vi "CalcTemp.vi"(8 "error in (no error)":errorcluster, 11 "S4GUI in":refnum<class "S4GUI.lvclass">) -> (0 "error out":errorcluster, 3 "S4GUI out":refnum<class "S4GUI.lvclass">)   [LabVIEW 2018, in "S4GUI.lvclass"]
uses:
  S4GUI.lvclass
  S4GUI.lvclass/S4GUI.ctl
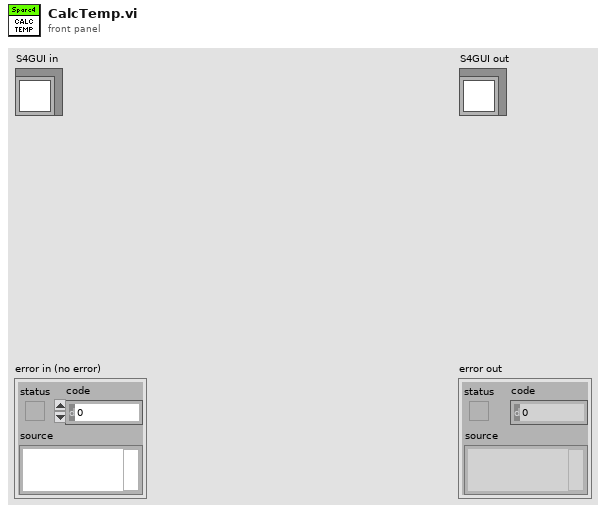
[diagram p1: front panel]
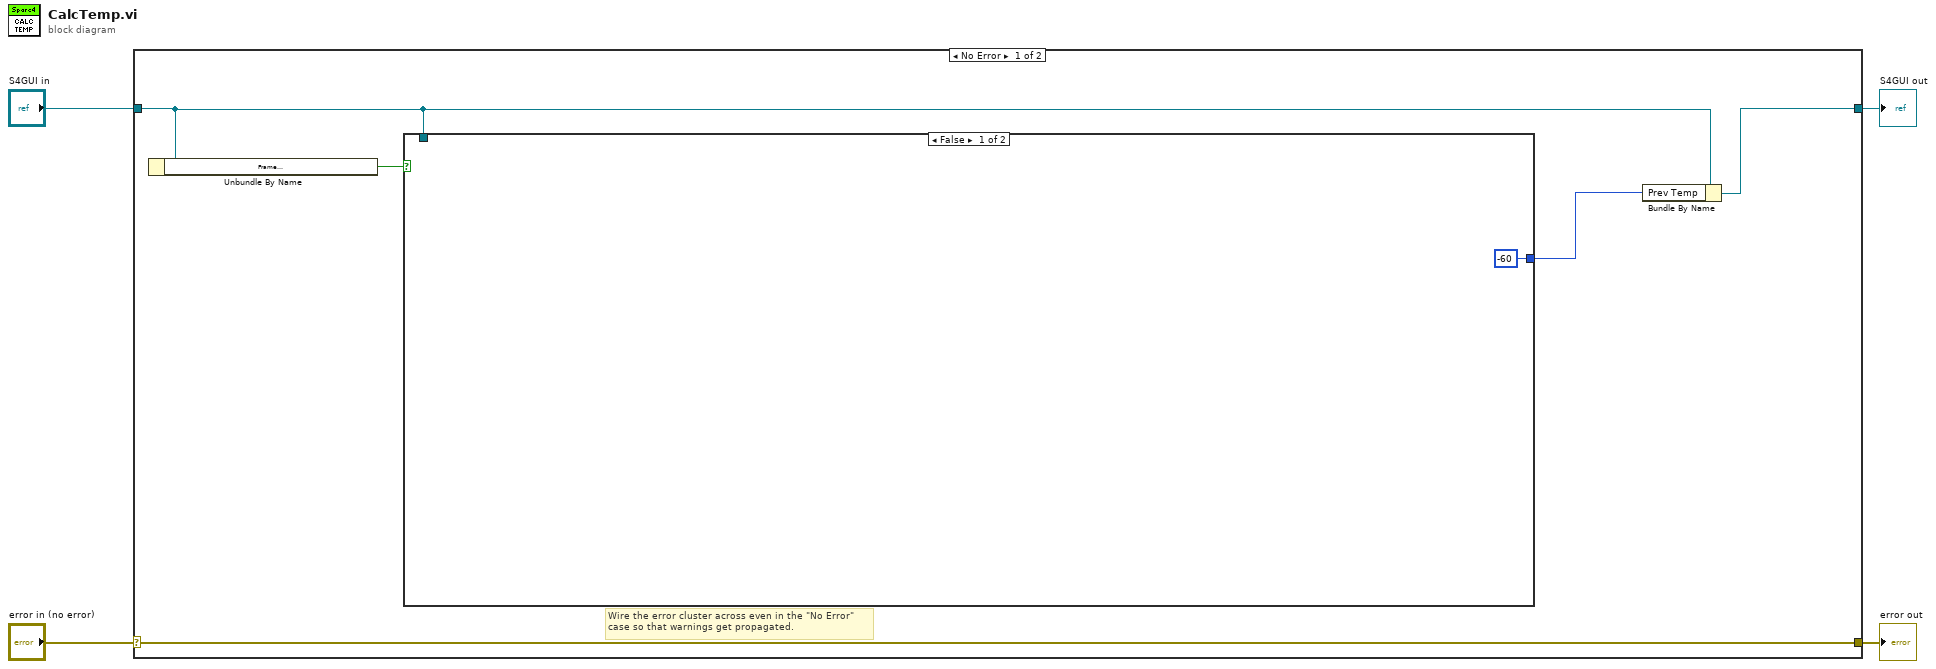
[diagram p0: block diagram]
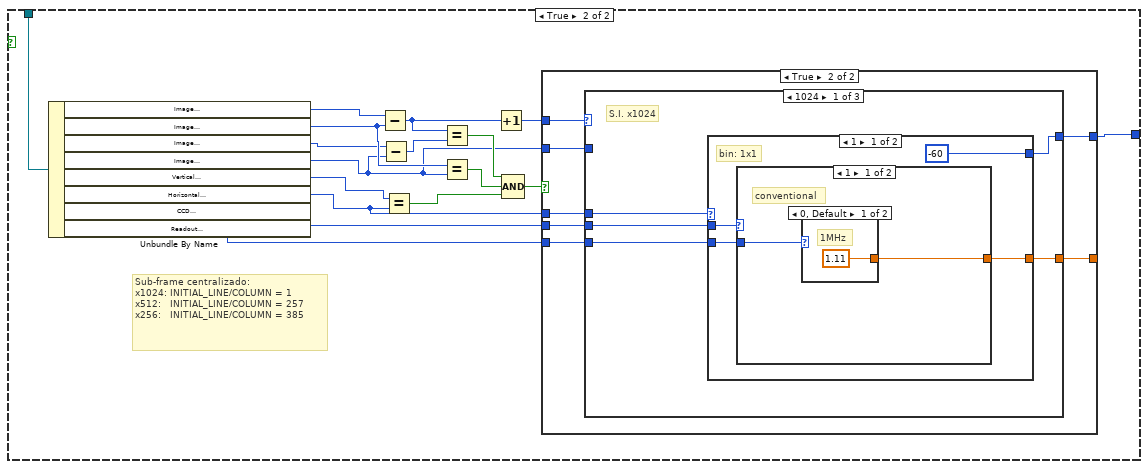
[diagram p2: hidden frame]
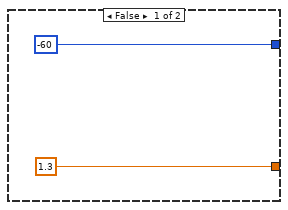
[diagram p3: hidden frame]
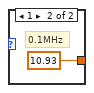
[diagram p4: hidden frame]
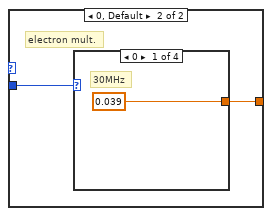
[diagram p5: hidden frame]
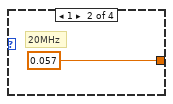
[diagram p6: hidden frame]
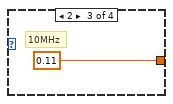
[diagram p7: hidden frame]
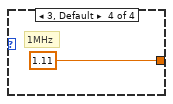
[diagram p8: hidden frame]
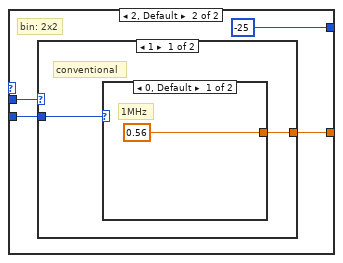
[diagram p9: hidden frame]
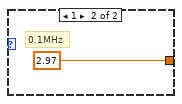
[diagram p10: hidden frame]
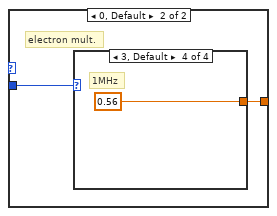
[diagram p11: hidden frame]
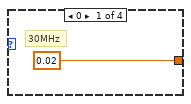
[diagram p12: hidden frame]
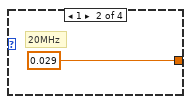
[diagram p13: hidden frame]
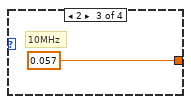
[diagram p14: hidden frame]
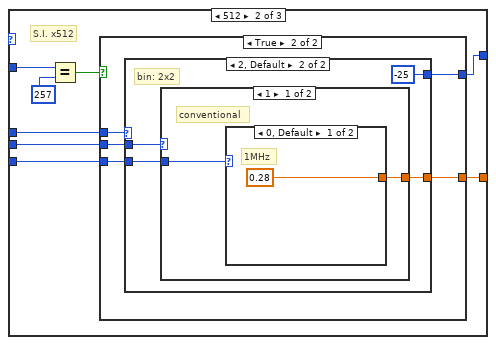
[diagram p15: hidden frame]
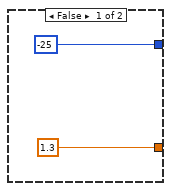
[diagram p16: hidden frame]
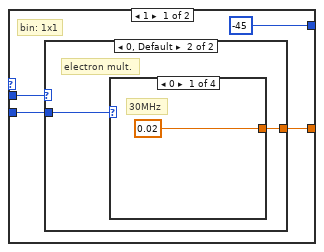
[diagram p17: hidden frame]
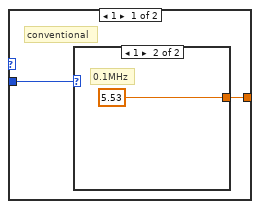
[diagram p18: hidden frame]
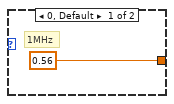
[diagram p19: hidden frame]
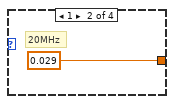
[diagram p20: hidden frame]
diagram:
  n1 = case shown="No Error" "error in (no error)" {
    selector: "error in (no error)" -> [w9 w157]
    tunnel: [w9 w157] -> w3
    tunnel: [w5 w156] -> w1
    tunnel: "S4GUI in" -> [w7 w156]
    frame No Error {
      # "Wire the error cluster across even in the \"No Error\"\ncase so that warnings get propagated."
      n2 = Unbundle By Name(w7) -> ("Frame\nTransfer"=w8:bool)
      n3 = case shown="False" w8 {
        tunnel: w7 -> [_ w27]
        tunnel: [i8 -60 ("y") w11] -> w6
        frame False {
        }
        frame True {
          # "Sub-frame centralizado:\nx1024: INITIAL_LINE/COLUMN = 1\nx512:   INITIAL_LINE/COLUMN = 257\nx256:   INITIAL_LINE/COLUMN = 385"
          n4 = Unbundle By Name(w27) -> ("Image\nFInal Column"=w19:u16, "Image\nInitial Column"=w18:u16, "Image\nFinal Line"=w17:u16, "Image \nInitial Line"=w16:u16, "Vertical\nBinning"=w15:u16, "Horizontal\nBinning"=w14:u16, "CCD \nEM Mode"=w13:u8, "Readout\nRate"=w12:u8)
          n5 = Subtract(x=w19, y=w18) -> (x-y=w23:u16)
          n6 = Subtract(x=w17, y=w16) -> (x-y=w20:u16)
          n7 = Equal?(x=w15, y=w14) -> (x = y?=w22:bool)
          n8 = Equal?(x=w23, y=w20) -> (x = y?=w25:bool)
          n9 = Equal?(x=w18, y=w16) -> (x = y?=w26:bool)
          n10 = Increment(x=w23) -> (x+1=w24:u16)
          n11 = Compound Arithmetic op=AND(w25, w26, w22) -> (w21:bool)
          n12 = case shown="True" w21 {
            tunnel: [1.3 ("y") w36] -> _
            tunnel: w13 -> [_ w35]
            tunnel: w12 -> [_ w34]
            tunnel: w24 -> [_ w33]
            tunnel: w14 -> [_ w32]
            tunnel: [i8 -60 ("y") w31] -> w11
            tunnel: w16 -> [_ w30]
            frame False {
            }
            frame True {
              n13 = case shown="1024" w33 {
                tunnel: [w41 w77 w120] -> w36
                tunnel: w35 -> [w40 w76 w119]
                tunnel: w34 -> [w39 w75 w118]
                tunnel: w32 -> [w38 w74 w117]
                tunnel: [w37 w73 w116] -> w31
                tunnel: w30 -> [_ w72 w114]
                frame 1024 {
                  # "S.I. x1024"
                  n14 = case shown="1" w38 {
                    tunnel: [w45 w59] -> w41
                    tunnel: w40 -> [w44 w58]
                    tunnel: w39 -> [w43 w57]
                    tunnel: [i8 -60 ("y") i8 -25 ("y")] -> w37
                    frame 1 {
                      # "bin: 1x1"
                      n15 = case shown="1" w44 {
                        tunnel: [w47 w51] -> w45
                        tunnel: w43 -> [w46 w50]
                        frame 1 {
                          # "conventional"
                          n16 = case shown="0, Default" w46 {
                            tunnel: [1.11 ("y") 10.93 ("y")] -> w47
                            frame 0, Default {
                              # "1MHz"
                            }
                            frame 1 {
                              # "0.1MHz"
                            }
                          }
                        }
                        frame 0, Default {
                          # "electron mult."
                          n17 = case shown="0" w50 {
                            tunnel: [0.039 ("y") 0.057 ("y") 0.11 ("y") 1.11 ("y")] -> w51
                            frame 0 {
                              # "30MHz"
                            }
                            frame 1 {
                              # "20MHz"
                            }
                            frame 2 {
                              # "10MHz"
                            }
                            frame 3, Default {
                              # "1MHz"
                            }
                          }
                        }
                      }
                    }
                    frame 2, Default {
                      # "bin: 2x2"
                      n18 = case shown="1" w58 {
                        tunnel: [w61 w65] -> w59
                        tunnel: w57 -> [w60 w64]
                        frame 1 {
                          # "conventional"
                          n19 = case shown="0, Default" w60 {
                            tunnel: [0.56 ("y") 2.97 ("y")] -> w61
                            frame 0, Default {
                              # "1MHz"
                            }
                            frame 1 {
                              # "0.1MHz"
                            }
                          }
                        }
                        frame 0, Default {
                          # "electron mult."
                          n20 = case shown="3, Default" w64 {
                            tunnel: [0.02 ("y") 0.029 ("y") 0.057 ("y") 0.56 ("y")] -> w65
                            frame 0 {
                              # "30MHz"
                            }
                            frame 1 {
                              # "20MHz"
                            }
                            frame 2 {
                              # "10MHz"
                            }
                            frame 3, Default {
                              # "1MHz"
                            }
                          }
                        }
                      }
                    }
                  }
                }
                frame 512 {
                  # "S.I. x512"
                  n21 = Equal?(x=w72, y=u16 257) -> (x = y?=w70:bool)
                  n22 = case shown="True" w70 {
                    tunnel: [1.3 ("y") w84] -> w77
                    tunnel: w76 -> [_ w83]
                    tunnel: w75 -> [_ w82]
                    tunnel: w74 -> [_ w81]
                    tunnel: [i8 -25 ("y") w80] -> w73
                    frame False {
                    }
                    frame True {
                      n23 = case shown="2, Default" w81 {
                        tunnel: [w88 w102] -> w84
                        tunnel: w83 -> [w87 w101]
                        tunnel: w82 -> [w86 w100]
                        tunnel: [i8 -45 ("y") i8 -25 ("y")] -> w80
                        frame 1 {
                          # "bin: 1x1"
                          n24 = case shown="0, Default" w87 {
                            tunnel: [w90 w94] -> w88
                            tunnel: w86 -> [w89 w93]
                            frame 1 {
                              # "conventional"
                              n25 = case shown="1" w89 {
                                tunnel: [0.56 ("y") 5.53 ("y")] -> w90
                                frame 0, Default {
                                # "1MHz"
                                }
                                frame 1 {
                                # "0.1MHz"
                                }
                              }
                            }
                            frame 0, Default {
                              # "electron mult."
                              n26 = case shown="0" w93 {
                                tunnel: [0.02 ("y") 0.029 ("y") 0.057 ("y") 0.56 ("y")] -> w94
                                frame 0 {
                                # "30MHz"
                                }
                                frame 1 {
                                # "20MHz"
                                }
                                frame 2 {
                                # "10MHz"
                                }
                                frame 3, Default {
                                # "1MHz"
                                }
                              }
                            }
                          }
                        }
                        frame 2, Default {
                          # "bin: 2x2"
                          n27 = case shown="1" w101 {
                            tunnel: [w104 w108] -> w102
                            tunnel: w100 -> [w103 w107]
                            frame 1 {
                              # "conventional"
                              n28 = case shown="0, Default" w103 {
                                tunnel: [0.28 ("y") 2.14 ("y")] -> w104
                                frame 0, Default {
                                # "1MHz"
                                }
                                frame 1 {
                                # "0.1MHz"
                                }
                              }
                            }
                            frame 0, Default {
                              # "electron mult."
                              n29 = case shown="3, Default" w107 {
                                tunnel: [0.011 ("y") 0.015 ("y") 0.029 ("y") 0.28 ("y")] -> w108
                                frame 0 {
                                # "30MHz"
                                }
                                frame 1 {
                                # "20MHz"
                                }
                                frame 2 {
                                # "10MHz"
                                }
                                frame 3, Default {
                                # "1MHz"
                                }
                              }
                            }
                          }
                        }
                      }
                    }
                  }
                }
                frame 256, Default {
                  # "S.I. x256"
                  n30 = Equal?(x=w114, y=u16 385) -> (x = y?=w113:bool)
                  n31 = case shown="True" w113 {
                    tunnel: [1.3 ("y") w127] -> w120
                    tunnel: w119 -> [_ w126]
                    tunnel: w118 -> [_ w125]
                    tunnel: w117 -> [_ w124]
                    tunnel: [i8 -10 ("y") w123] -> w116
                    frame False {
                    }
                    frame True {
                      n32 = case shown="1" w124 {
                        tunnel: [w131 w145] -> w127
                        tunnel: w126 -> [w130 w144]
                        tunnel: w125 -> [w129 w143]
                        tunnel: [i8 -33 ("y") i8 -10 ("y")] -> w123
                        frame 1 {
                          # "bin: 1x1"
                          n33 = case shown="0, Default" w130 {
                            tunnel: [w133 w137] -> w131
                            tunnel: w129 -> [w132 w136]
                            frame 1 {
                              # "conventional"
                              n34 = case shown="0, Default" w132 {
                                tunnel: [0.28 ("y") 2.79 ("y")] -> w133
                                frame 0, Default {
                                # "1MHz"
                                }
                                frame 1 {
                                # "0.1MHz"
                                }
                              }
                            }
                            frame 0, Default {
                              # "electron mult."
                              n35 = case shown="1" w136 {
                                tunnel: [0.011 ("y") 0.015 ("y") 0.029 ("y") 0.28 ("y")] -> w137
                                frame 0 {
                                # "30MHz"
                                }
                                frame 1 {
                                # "20MHz"
                                }
                                frame 2 {
                                # "10MHz"
                                }
                                frame 3, Default {
                                # "1MHz"
                                }
                              }
                            }
                          }
                        }
                        frame 2, Default {
                          # "bin: 2x2"
                          n36 = case shown="0, Default" w144 {
                            tunnel: [w147 w151] -> w145
                            tunnel: w143 -> [w146 w150]
                            frame 1 {
                              # "conventional"
                              n37 = case shown="0, Default" w146 {
                                tunnel: [0.14 ("y") 1.24 ("y")] -> w147
                                frame 0, Default {
                                # "1MHz"
                                }
                                frame 1 {
                                # "0.1MHz"
                                }
                              }
                            }
                            frame 0, Default {
                              # "electron mult."
                              n38 = case shown="3, Default" w150 {
                                tunnel: [0.0059 ("y") 0.0083 ("y") 0.015 ("y") 0.14 ("y")] -> w151
                                frame 0 {
                                # "30MHz"
                                }
                                frame 1 {
                                # "20MHz"
                                }
                                frame 2 {
                                # "10MHz"
                                }
                                frame 3, Default {
                                # "1MHz"
                                }
                              }
                            }
                          }
                        }
                      }
                    }
                  }
                }
              }
            }
          }
        }
      }
      n39 = Bundle By Name(cluster=w7, "Prev Temp"=w6) -> (w5:refnum<class "S4GUI.lvclass">)
    }
    frame Error {
    }
  }
  "error out" <- w3
  "S4GUI out" <- w1
